vi "while循环的使用(下).vi"() -> ()   [LabVIEW 2018]
panel:
  out "字符串 2":string
  in  "字符串":string
  out "数值 2":i32
  out "数值":i32
  out "x+1":i32
  in  "停止":bool
  # "1+2+3+...+100"
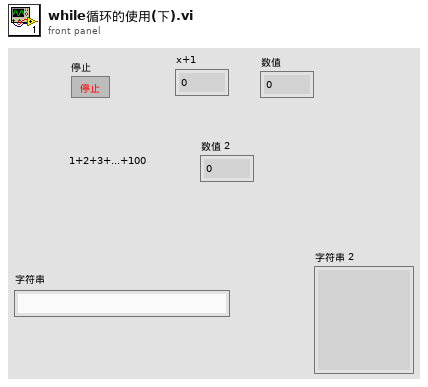
[diagram p1: front panel]
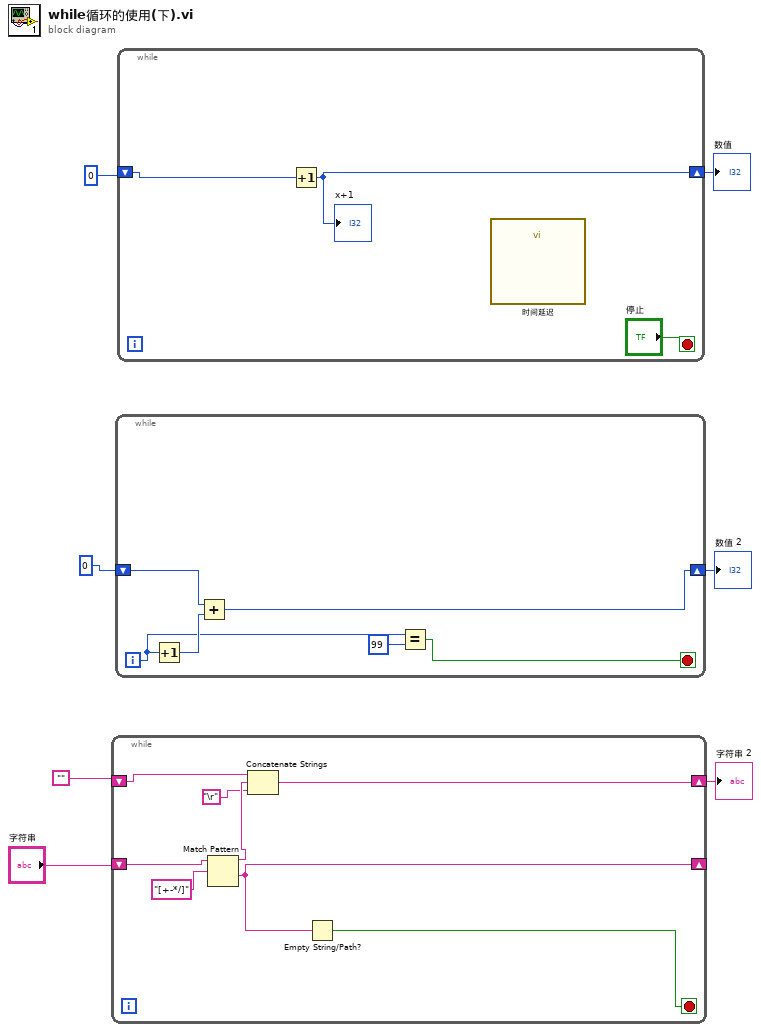
[diagram p0: block diagram]
diagram:
  n1 = while {
    shift-right: [w9] -> _
    shift-left: "字符串" -> [w15]
    shift-right: [w10] -> w1
    shift-left: "" -> [w13]
    stop <- w8 stop-if-true
    n2 = Match Pattern(string=w15, regular expression="[+-*/]" ("正则表达式")) -> (before substring=w12:string, after substring=w9:string)  [unwired: 1 in, 2 out]
    n3 = Concatenate Strings(w13, w12, "\r") -> (w10:string)
    n4 = Empty String/Path?(string/path=w9) -> (empty?=w8:bool)
  }
  "字符串 2" <- w1
  n5 = while {
    shift-right: [w19] -> w4
    shift-left: 0 -> [w20]
    i -> [w18]
    stop <- w16 stop-if-true
    n6 = Increment(x=w18) -> (x+1=w21:i32)
    n7 = Add(x=w20, y=w21) -> (x+y=w19:i32)
    n8 = Equal?(x=w18, y=99) -> (x = y?=w16:bool)
  }
  "数值 2" <- w4
  n9 = while {
    shift-right: [w22] -> w6
    shift-left: 0 -> [w23]
    stop <- "停止" stop-if-true
    n10 = Increment(x=w23) -> (x+1=w22:i32)
    "x+1" <- w22
    n11 = call "时间延迟"() -> ()  [unwired: 11 in, 1 out]
  }
  "数值" <- w6
